vi "Tektronix.vi"(7 "JPG":refnum<vi>, 11 "Console Reference":refnum<vi>) -> ()   [LabVIEW 2022 SP3]
panel:
  in  "stop":bool
  out "plot":cluster{dbl, dbl, dbl[]}(graph)
  in  "VISA":refnum<visa-resource-name>
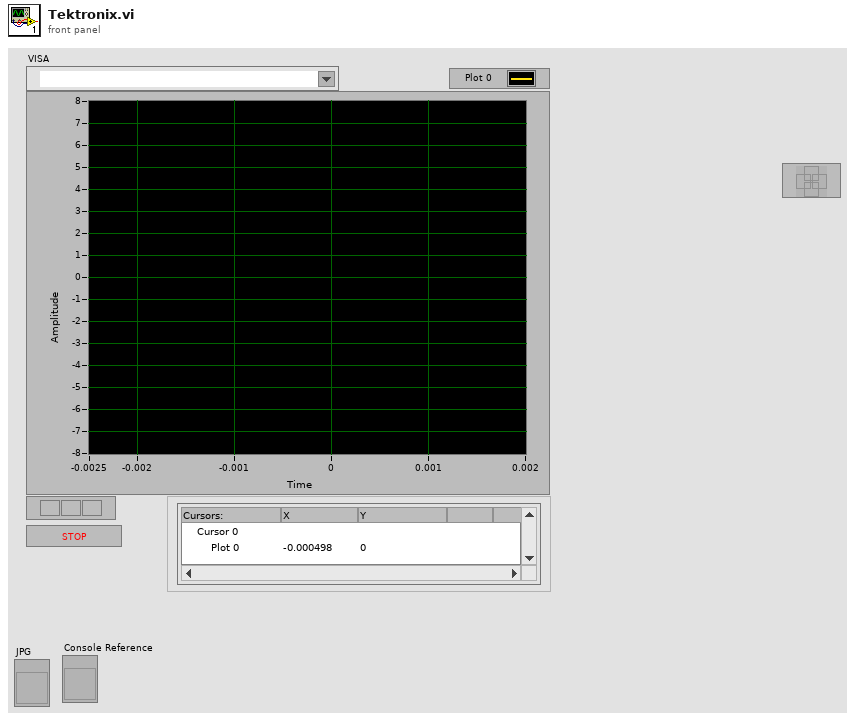
[diagram p1: front panel]
types:
  T1 = enum8{"Enabled", "Disabled", "Disabled and Grayed Out"}
  T2 = cluster{"Xmax":dbl, "Xmin":dbl, "Ymax":dbl, "Ymin":dbl}
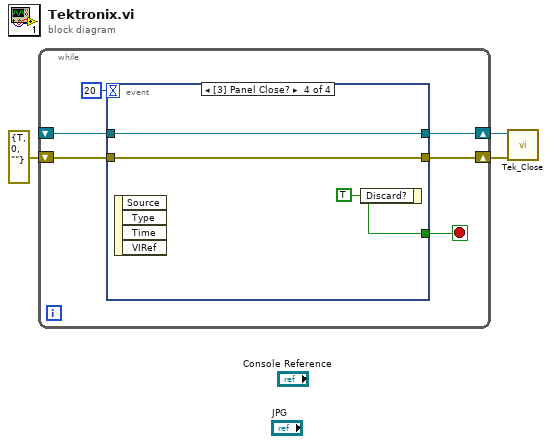
[diagram p0: block diagram]
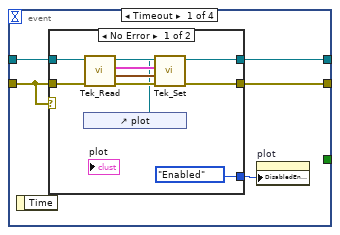
[diagram p2: hidden frame]
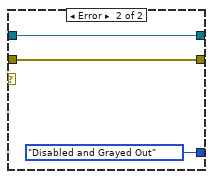
[diagram p3: hidden frame]
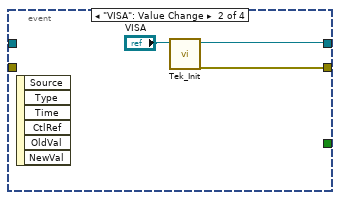
[diagram p4: hidden frame]
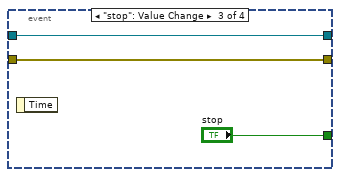
[diagram p5: hidden frame]
diagram:
  n1 = while {
    shift-right: [w9] -> w3
    shift-left: _ -> [w8]
    shift-right: [w6] -> w2
    shift-left: errorcluster {"status"=TRUE, "code"=0, "source"=""} ("error out") -> [w7]
    stop <- w5 stop-if-true
    n2 = event shown="[3] Panel Close?" {
      selector: _ -> [_ _ _ _]
      dyn-events: _ -> [_ _ _ _]
      timeout: 20 -> [_ _ _ _]
      tunnel: [w14 "VISA" w29 w33] -> w9
      tunnel: w8 -> [w13 _ w29 w33]
      tunnel: w7 -> [w11 _ w28 w32]
      tunnel: [w12 w27 w28 w32] -> w6
      tunnel: [_ _ "stop" w31] -> w5
      event Timeout {
        n3 = event-data() -> ()  [unwired: 1 in, 1 out]
        n4 = case shown="No Error" w11 {
          tunnel: [w22 w25] -> w14
          tunnel: w13 -> [w21 w25]
          tunnel: w11 -> [w20 w24]
          tunnel: [w19 w24] -> w12
          tunnel: [T1."Enabled" ("Disabled") T1."Disabled and Grayed Out" ("Disabled")] -> w10
          frame No Error {
            n5 = control-ref of="plot"() -> (w15:refnum<vi>)
            n6 = call "Tek_Read.vi"("error in (no error)"=w20, "VISA Refnum in"=w21) -> ("error out"=w19:errorcluster, "range"=w16:T2, "Scope"=w17:cluster{dbl, dbl, dbl[]}, "VISA Refnum out"=w22:refnum<visa-resource-name>)  [unwired: 6 in]
            n7 = call "Tek_Set.vi"("error in (no error)"=w19, "range"=w16, "Scope"=w17, "plot"=w15) -> ()  [unwired: 8 in]
          }
          frame Error {
          }
        }
        n8 = property on="plot" class="WFGraph (strict)"("DisabledEnum"=w10) -> ()  [unwired: 2 in, 2 out]
      }
      event "VISA": Value Change {
        n9 = event-data() -> ()  [unwired: 1 in, 6 out]
        n10 = call "Tek_Init.vi"("VISA"="VISA") -> ("error out"=w27:errorcluster)  [unwired: 9 in, 1 out]
      }
      event "stop": Value Change {
        n11 = event-data() -> ()  [unwired: 1 in, 1 out]
      }
      event Panel Close? {
        w31 = TRUE ("Discard?")
        n12 = event-data() -> ()  [unwired: 1 in, 4 out]
        n13 = event-data("Discard?"=w31) -> ()  [unwired: 1 in, 1 out]
      }
    }
  }
  n14 = call "Tek_Close.vi"("error in (no error)"=w2, "VISA Refnum in"=w3) -> ()  [unwired: 10 in]
